vi "Demo.vi"() -> ()   [LabVIEW 2020]
uses:
  <vilib>/ErrorRing/Error Ring.xnode
  <vilib>/Utility/error.llb/Error Cluster From Error Code.vi
  <vilib>/security/Message Digest/API/NI_Message Digest API.lvlib
  4385dd5b-b65c-4a35-88a7-d4638a257287.vi
  c83e9a0e-abd6-4d9c-830f-6cf58d083650.vi
  <vilib>/Utility/Data Type/NI_Data Type.lvlib
  <vilib>/MultiError/TokenizeJSON/Multi Error Cluster.lvlib
  <vilib>/security/Message Digest/API/Instances/Byte Array/SHA-256 Byte Array Checksum.vi
panel:
  in  "Text Ring":u16(ring) items=["Done This ", "Done That", "Working on This"]
  out "array of errors":errorcluster[](array[cluster])
  out "array of enums":enum16{"Item 1", "Item 2", "Item 3"}[](array[ring])
  out "maximum value for type":fxp<+,4,4>
  out "minimum value for type":fxp<+,4,4>
  out "NI GUID":string
  out "total physical memory":u64
  out "memory allocated for LabVIEW":u64
  out "free physical memory":u64
  out "Data Compromised?":bool
  out "digest":string
  out "error out":errorcluster
  out "Array":string[](array[string])
  out "concatenated string":string
  out "x+y":dbl
  in  "x":dbl
  in  "y":dbl
  out "Variant Indicator":variant=variant(string "Oh NO!\nThis is some data in a varient!")
  in  "Variant Control":variant=variant(string "Oh NO!\nThis is some data in a varient!")
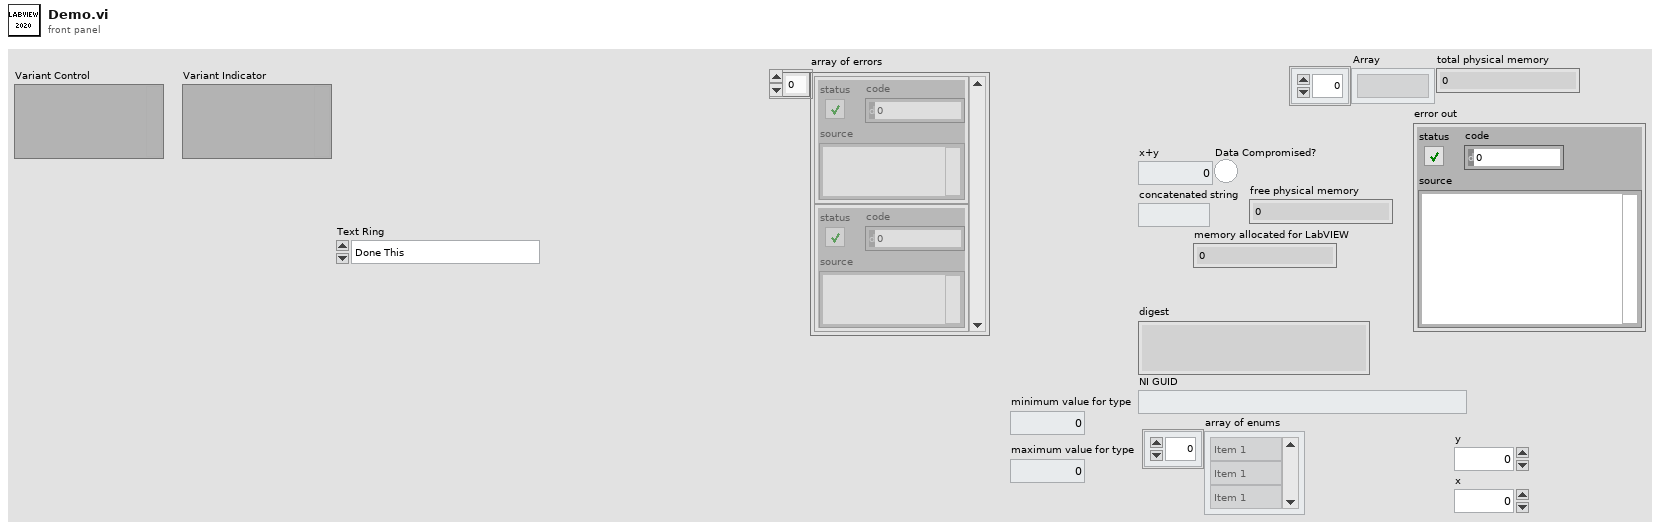
[diagram p1: front panel]
types:
  T1 = enum16{"Item: 0", "Item: 1", "Item: 2", "Item: 3", "Item: 4", "Item: 5", "Item: 6", "Item: 7", "Item: 8", "Item: 9", "Item: 10", "Item: 11", "Item: 12", "Item: 13", "Item: 14", "Item: 15", "Item: 16", "Item: 17", "Item: 18", "Item: 19", "Item: 20", "Item: 21", "Item: 22", "Item: 23", "Item: 24", "Item: 25", "Item: 26", "Item: 27", "Item: 28", "Item: 29", "Item: 30", "Item: 31", "Item: 32", "Item: 33", "Item: 34", "Item: 35", "Item: 36", "Item: 37", "Item: 38", "Item: 39", "Item: 40", "Item: 41", "Item: 42", "Item: 43", "Item: 44", "Item: 45", "Item: 46", "Item: 47", "Item: 48", "Item: 49", "Item: 50", "Item: 51", "Item: 52", "Item: 53", "Item: 54", "Item: 55", "Item: 56", "Item: 57", "Item: 58", "Item: 59", "Item: 60", "Item: 61", "Item: 62", "Item: 63", "Item: 64", "Item: 65", "Item: 66", "Item: 67", "Item: 68", "Item: 69", "Item: 70", "Item: 71", "Item: 72", "Item: 73", "Item: 74", "Item: 75", "Item: 76", "Item: 77", "Item: 78", "Item: 79", "Item: 80", "Item: 81", "Item: 82", "Item: 83", "Item: 84", "Item: 85", "Item: 86", "Item: 87", "Item: 88", "Item: 89", "Item: 90", "Item: 91", "Item: 92", "Item: 93", "Item: 94", "Item: 95", "Item: 96", "Item: 97", "Item: 98", "Item: 99"}
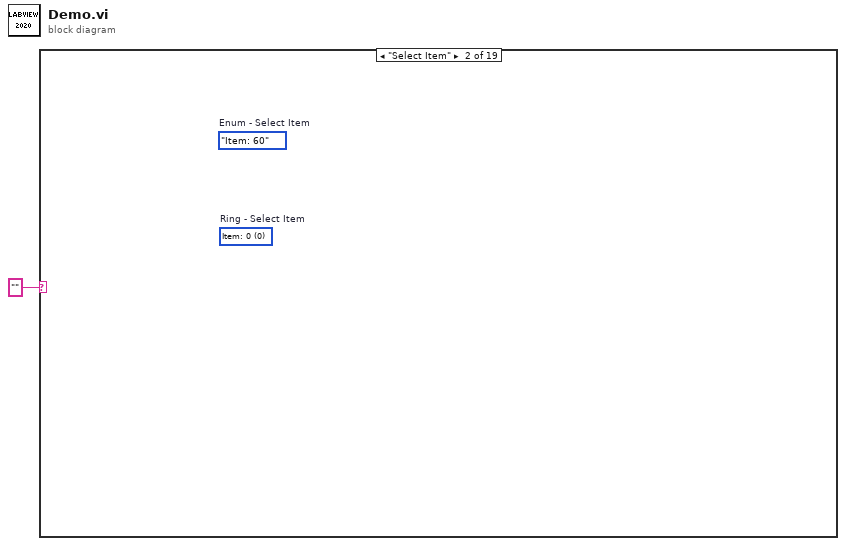
[diagram p0: block diagram]
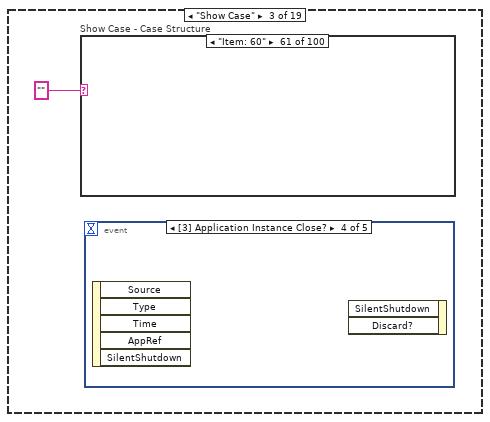
[diagram p3: hidden frame]
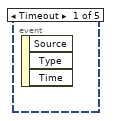
[diagram p4: hidden frame]
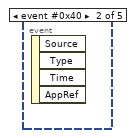
[diagram p5: hidden frame]
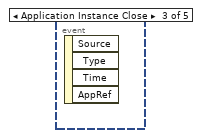
[diagram p6: hidden frame]
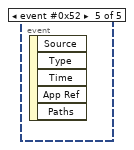
[diagram p7: hidden frame]
diagram:
  n1 = case shown="\"Select Item\"" "" {
    frame Default {
    }
    frame "Select Item" {
      (unwired) u16 0 items=["Item: 0", "Item: 1", "Item: 2", "Item: 3", "Item: 4", "Item: 5", "Item: 6", "Item: 7", "Item: 8", "Item: 9", "Item: 10", "Item: 11", "Item: 12", "Item: 13", "Item: 14", "Item: 15", "Item: 16", "Item: 17", "Item: 18", "Item: 19", "Item: 20", "Item: 21", "Item: 22", "Item: 23", "Item: 24", "Item: 25", "Item: 26", "Item: 27", "Item: 28", "Item: 29", "Item: 30", "Item: 31", "Item: 32", "Item: 33", "Item: 34", "Item: 35", "Item: 36", "Item: 37", "Item: 38", "Item: 39", "Item: 40", "Item: 41", "Item: 42", "Item: 43", "Item: 44", "Item: 45", "Item: 46", "Item: 47", "Item: 48", "Item: 49", "Item: 50", "Item: 51", "Item: 52", "Item: 53", "Item: 54", "Item: 55", "Item: 56", "Item: 57", "Item: 58", "Item: 59", "Item: 60", "Item: 61", "Item: 62", "Item: 63", "Item: 64", "Item: 65", "Item: 66", "Item: 67", "Item: 68", "Item: 69", "Item: 70", "Item: 71", "Item: 72", "Item: 73", "Item: 74", "Item: 75", "Item: 76", "Item: 77", "Item: 78", "Item: 79", "Item: 80", "Item: 81", "Item: 82", "Item: 83", "Item: 84", "Item: 85", "Item: 86", "Item: 87", "Item: 88", "Item: 89", "Item: 90", "Item: 91", "Item: 92", "Item: 93", "Item: 94", "Item: 95", "Item: 96", "Item: 97", "Item: 98", "Item: 99"]  # Ring - Select Item
      (unwired) T1."Item: 60"  # Enum - Select Item
    }
    frame "Show Case" {
      n2 = case "Show Case - Case Structure" shown="\"Item: 60\"" "" {
        frame "Item: 0", Default {
        }
        frame "Item: 1" {
        }
        frame "Item: 2" {
        }
        frame "Item: 3" {
        }
        frame "Item: 4" {
        }
        frame "Item: 5" {
        }
        frame "Item: 6" {
        }
        frame "Item: 7" {
        }
        frame "Item: 8" {
        }
        frame "Item: 9" {
        }
        frame "Item: 10" {
        }
        frame "Item: 11" {
        }
        frame "Item: 12" {
        }
        frame "Item: 13" {
        }
        frame "Item: 14" {
        }
        frame "Item: 15" {
        }
        frame "Item: 16" {
        }
        frame "Item: 17" {
        }
        frame "Item: 18" {
        }
        frame "Item: 19" {
        }
        frame "Item: 20" {
        }
        frame "Item: 21" {
        }
        frame "Item: 22" {
        }
        frame "Item: 23" {
        }
        frame "Item: 24" {
        }
        frame "Item: 25" {
        }
        frame "Item: 26" {
        }
        frame "Item: 27" {
        }
        frame "Item: 28" {
        }
        frame "Item: 29" {
        }
        frame "Item: 30" {
        }
        frame "Item: 31" {
        }
        frame "Item: 32" {
        }
        frame "Item: 33" {
        }
        frame "Item: 34" {
        }
        frame "Item: 35" {
        }
        frame "Item: 36" {
        }
        frame "Item: 37" {
        }
        frame "Item: 38" {
        }
        frame "Item: 39" {
        }
        frame "Item: 40" {
        }
        frame "Item: 41" {
        }
        frame "Item: 42" {
        }
        frame "Item: 43" {
        }
        frame "Item: 44" {
        }
        frame "Item: 45" {
        }
        frame "Item: 46" {
        }
        frame "Item: 47" {
        }
        frame "Item: 48" {
        }
        frame "Item: 49" {
        }
        frame "Item: 50" {
        }
        frame "Item: 51" {
        }
        frame "Item: 52" {
        }
        frame "Item: 53" {
        }
        frame "Item: 54" {
        }
        frame "Item: 55" {
        }
        frame "Item: 56" {
        }
        frame "Item: 57" {
        }
        frame "Item: 58" {
        }
        frame "Item: 59" {
        }
        frame "Item: 60" {
        }
        frame "Item: 61" {
        }
        frame "Item: 62" {
        }
        frame "Item: 63" {
        }
        frame "Item: 64" {
        }
        frame "Item: 65" {
        }
        frame "Item: 66" {
        }
        frame "Item: 67" {
        }
        frame "Item: 68" {
        }
        frame "Item: 69" {
        }
        frame "Item: 70" {
        }
        frame "Item: 71" {
        }
        frame "Item: 72" {
        }
        frame "Item: 73" {
        }
        frame "Item: 74" {
        }
        frame "Item: 75" {
        }
        frame "Item: 76" {
        }
        frame "Item: 77" {
        }
        frame "Item: 78" {
        }
        frame "Item: 79" {
        }
        frame "Item: 80" {
        }
        frame "Item: 81" {
        }
        frame "Item: 82" {
        }
        frame "Item: 83" {
        }
        frame "Item: 84" {
        }
        frame "Item: 85" {
        }
        frame "Item: 86" {
        }
        frame "Item: 87" {
        }
        frame "Item: 88" {
        }
        frame "Item: 89" {
        }
        frame "Item: 90" {
        }
        frame "Item: 91" {
        }
        frame "Item: 92" {
        }
        frame "Item: 93" {
        }
        frame "Item: 94" {
        }
        frame "Item: 95" {
        }
        frame "Item: 96" {
        }
        frame "Item: 97" {
        }
        frame "Item: 98" {
        }
        frame "Item: 99" {
        }
      }
      n3 = event shown="[3] Application Instance Close?" {
        selector: _ -> [_ _ _ _ _]
        dyn-events: _ -> [_ _ _ _ _]
        timeout: _ -> [_ _ _ _ _]
        event Timeout {
          n4 = event-data() -> ()  [unwired: 1 in, 3 out]
        }
        event event #0x40 {
          n5 = event-data() -> ()  [unwired: 1 in, 4 out]
        }
        event Application Instance Close {
          n6 = event-data() -> ()  [unwired: 1 in, 4 out]
        }
        event Application Instance Close? {
          n7 = event-data() -> ()  [unwired: 1 in, 5 out]
          n8 = event-data() -> ()  [unwired: 3 in, 1 out]
        }
        event event #0x52 {
          n9 = event-data() -> ()  [unwired: 1 in, 5 out]
        }
      }
    }
    frame "Rearranging Cases" {
      n10 = case "Rearrange - Case Structure" shown="\"Item: 0\", Default" "" {
        frame "Item: 0", Default {
        }
        frame "Item: 1" {
        }
        frame "Item: 10" {
        }
        frame "Item: 11" {
        }
        frame "Item: 12" {
        }
        frame "Item: 13" {
        }
        frame "Item: 14" {
        }
        frame "Item: 15" {
        }
        frame "Item: 16" {
        }
        frame "Item: 17" {
        }
        frame "Item: 18" {
        }
        frame "Item: 19" {
        }
        frame "Item: 2" {
        }
        frame "Item: 20" {
        }
        frame "Item: 21" {
        }
        frame "Item: 22" {
        }
        frame "Item: 23" {
        }
        frame "Item: 24" {
        }
        frame "Item: 25" {
        }
        frame "Item: 26" {
        }
        frame "Item: 27" {
        }
        frame "Item: 28" {
        }
        frame "Item: 29" {
        }
        frame "Item: 3" {
        }
        frame "Item: 30" {
        }
        frame "Item: 31" {
        }
        frame "Item: 32" {
        }
        frame "Item: 33" {
        }
        frame "Item: 34" {
        }
        frame "Item: 35" {
        }
        frame "Item: 36" {
        }
        frame "Item: 37" {
        }
        frame "Item: 38" {
        }
        frame "Item: 39" {
        }
        frame "Item: 4" {
        }
        frame "Item: 40" {
        }
        frame "Item: 41" {
        }
        frame "Item: 42" {
        }
        frame "Item: 43" {
        }
        frame "Item: 44" {
        }
        frame "Item: 45" {
        }
        frame "Item: 46" {
        }
        frame "Item: 47" {
        }
        frame "Item: 48" {
        }
        frame "Item: 49" {
        }
        frame "Item: 5" {
        }
        frame "Item: 50" {
        }
        frame "Item: 51" {
        }
        frame "Item: 52" {
        }
        frame "Item: 53" {
        }
        frame "Item: 54" {
        }
        frame "Item: 55" {
        }
        frame "Item: 56" {
        }
        frame "Item: 57" {
        }
        frame "Item: 58" {
        }
        frame "Item: 59" {
        }
        frame "Item: 6" {
        }
        frame "Item: 60" {
        }
        frame "Item: 61" {
        }
        frame "Item: 62" {
        }
        frame "Item: 63" {
        }
        frame "Item: 64" {
        }
        frame "Item: 7" {
        }
        frame "Item: 73" {
        }
        frame "Item: 74" {
        }
        frame "Item: 75" {
        }
        frame "Item: 76" {
        }
        frame "Item: 77" {
        }
        frame "Item: 78" {
        }
        frame "Item: 79" {
        }
        frame "Item: 8" {
        }
        frame "Item: 80" {
        }
        frame "Item: 81" {
        }
        frame "Item: 82" {
        }
        frame "Item: 83" {
        }
        frame "Item: 84" {
        }
        frame "Item: 85" {
        }
        frame "Item: 86" {
        }
        frame "Item: 87" {
        }
        frame "Item: 88" {
        }
        frame "Item: 89" {
        }
        frame "Item: 9" {
        }
        frame "Item: 90" {
        }
        frame "Item: 91" {
        }
        frame "Item: 92" {
        }
        frame "Item: 93" {
        }
        frame "Item: 94" {
        }
        frame "Item: 95" {
        }
        frame "Item: 96" {
        }
        frame "Item: 97" {
        }
        frame "Item: 98" {
        }
        frame "Item: 99" {
        }
      }
      n11 = event shown="[0] Timeout" {
        selector: _ -> [_ _ _ _ _]
        dyn-events: _ -> [_ _ _ _ _]
        timeout: _ -> [_ _ _ _ _]
        event Timeout {
          n12 = event-data() -> ()  [unwired: 1 in, 3 out]
        }
        event event #0x40 {
          n13 = event-data() -> ()  [unwired: 1 in, 4 out]
        }
        event Application Instance Close {
          n14 = event-data() -> ()  [unwired: 1 in, 4 out]
        }
        event Application Instance Close? {
          n15 = event-data() -> ()  [unwired: 1 in, 5 out]
          n16 = event-data() -> ()  [unwired: 3 in, 1 out]
        }
        event event #0x52 {
          n17 = event-data() -> ()  [unwired: 1 in, 5 out]
        }
      }
    }
    frame "Clear Varient" {
      (unwired) variant(string "Oh NO!\nThis is some data in a varient!") ("Variant")
    }
    frame "Root Cause" {
      n18 = call "Broken VI.vi"() -> ()  [unwired: 12 in]
    }
    frame "Cluster Size" {
      n19 = Array To Cluster(array=bool[] []) -> ()  [unwired: 1 out]
    }
    frame "Last Item in Ring" {
      n20 = property on="Text Ring" class="Ring (strict)" props=["Last Value Hidden"]() -> ()  [unwired: 2 in, 3 out]
    }
    frame "Clean up broken wires" {
      n21 = Add(x="x", y="y") -> (x+y=→"x+y":dbl)
      n22 = Concatenate Strings("Concatenate String with Float" ("string")) -> (→"concatenated string":string)
    }
    frame "Hide Event Node" {
      n23 = event shown="[3] Menu Selection? (App)" {
        selector: _ -> [_ _ _ _]
        dyn-events: _ -> [_ _ _ _]
        timeout: _ -> [_ _ _ _]
        event Timeout {
          n24 = event-data() -> ()  [unwired: 1 in, 3 out]
        }
        event Panel Close? {
          n25 = event-data() -> ()  [unwired: 1 in, 4 out]
          n26 = event-data() -> ()  [unwired: 2 in, 1 out]
        }
        event Menu Selection (App) {
          n27 = event-data() -> ()  [unwired: 1 in, 7 out]
        }
        event Menu Selection? (App) {
          n28 = event-data() -> ()  [unwired: 1 in, 1 out]
          n29 = event-data() -> ()  [unwired: 2 in, 1 out]
        }
      }
    }
    frame "Iteration Terminal" {
      w10 = map{string, i32} {}  # Size: 0
      n30 = for {
        tunnel: w10 -> [w12] mode=indexing
        tunnel: [w11] -> _ mode=indexing
        n31 = Unbundle(w12) -> (w11:string)  [unwired: 1 out]
      }
    }
    frame "Swapping Wires" {
      n32 = Add(x=0.0) -> ()  [unwired: 1 in, 1 out]
    }
    frame "Change icon" {
      n33 = call "Change the icon.vi"() -> ()  [unwired: 12 in]
    }
    frame "Insert Function" {
      n34 = Insert Into Array(array=string[] []) -> (→"Array":string[])  [unwired: 2 in]
    }
    frame "Quick Drop Context Help" {
    }
    frame "Multiple Errors" {
      (unwired) errorcluster {"status"=TRUE, "code"=-2147483638, "source"="<JSONErrorSingle_1.0>{\n    \"status\": true,\n    \"code\": -2147483638,\n    \"source\": \"Demo.vi<APPEND>\\n\\n<b>Complete call chain:</b>\\r\\n     Demo.vi\"\n,\"attributes\":[{\"Attribute 1\":Value 1}]}"} ("error out")
      n35 = xnode "Error Ring"() -> ("error out"=w16:errorcluster)
      n36 = xnode "Error Ring"() -> ("error out"=w18:errorcluster)
      n37 = Merge Errors(w16, w18) -> (w19:errorcluster)
      "error out" <- w19
      n38 = call <vilib>:"Error Cluster to Array of Errors.vi"("error"=w19) -> ("array of errors"=→"array of errors":errorcluster[])  [unwired: 10 in]
    }
    frame "Transport Layer Security" {
    }
    frame "digest" {
      # "Project provider ini file example of hashing (one-way cryptography)"
      # "[Provider]\nSupportedType={D60740D6-F254-4BBC-5675-8858F35B810E}\nSupportedType={D60740D6-F254-4BBC-5675-8858F35B820E}\nSupportedType={ABC740D6-F254-4BBC-5675-8858F35B820E}\nSupportedType={EFD740D6-F254-4BBC-5675-8858F35B820E}\nGlobalItemInterfaceVI=..\\TomsToolsDocumentationTool\\TomsToolsDocumentationTool_Global_Interface.vi\nItemInterfaceVI=..\\TomsToolsDocumentationTool\\TomsToolsDocumentationTool_Item_Interface.vi\nProviderInterfaceVI=..\\TomsToolsDocumentationTool\\TomsToolsDocumentationTool_Provider_Interface.vi\nIsPrimary=0\nLicenseName=None\nInterfaceVersion=1.0\nSignature=N2LBC33C33NK9K9C5SWNW773JC79SCXB"
      n39 = call-poly <vilib>:"Byte Array Checksum.vi"("buffer"=u8[] [123, 45, 87]) -> ("digest"=w30:string)  [unwired: 10 in]
      "digest" <- w30
      n40 = Not Equal?(x="9163ffcb247b0034748ae017bcc96bcbb13c7194fa0e042e9bbef7e9c50438c9" ("digest"), y=w30) -> (x != y?=→"Data Compromised?":bool)
    }
    frame "New Functions" {
      (unwired) enum16{"Item 1", "Item 2", "Item 3"}[] [enum."Item 1", enum."Item 2", enum."Item 3"] items=["Item 1", "Item 2", "Item 3"] ("array of enums")
      (unwired) 0
      (unwired) 0.0
      w37 = fxp<+,4,4> 0.0  # Fixed Point (+,4,4)
      (unwired) "1004AA72-2F99-4B9E-84E3-FBDE15714653" ("NI GUID")
      # "Returns\nGlobally Unique Identifier (GUID)"
      n41 = call <vilib>:"Get Memory Status.vi"() -> ("free physical memory"=→"free physical memory":u64, "memory allocated for LabVIEW"=→"memory allocated for LabVIEW":u64, "total physical memory"=→"total physical memory":u64)  [unwired: 8 in, 1 out]
      n42 = call "Range Limits for Type.vim"("type"=w37) -> ("minimum value for type"=→"minimum value for type":fxp<+,4,4>, "maximum value for type"=→"maximum value for type":fxp<+,4,4>)  [unwired: 9 in]
      n43 = call <vilib>:"Get LabVIEW Class Parent And Member VI Information.vi"("variant"=variant) -> ()  [unwired: 7 in, 4 out]
      n44 = call <vilib>:"Create NI GUID.vi"() -> ("NI GUID"=→"NI GUID":string)
      n45 = call "Enum to Array of Enums.vim"("enum"=enum16{"Item 1", "Item 2", "Item 3"}."Item 1") -> ("array of enums"=w33:enum16{"Item 1", "Item 2", "Item 3"}[])
      "array of enums" <- w33
      n46 = for {
        tunnel: w33 -> [w42] mode=indexing
        n47 = case shown="\"Item 2\"" w42 {
          frame "Item 1", Default {
          }
          frame "Item 2" {
          }
          frame "Item 3" {
          }
        }
      }
    }
  }
